vi "SOUR_POW_ALC_MODE_CAT.vi"(0 "VISA IN":refnum<visa-resource-name>, 1 "Port number":i32, 2 "Source Port":string, 5 "error in":errorcluster, 7 "Channel":i32) -> (14 "VISA Out":refnum<visa-resource-name>, 16 "Data":string, 19 "error out":errorcluster)   [LabVIEW 2018, in "PNA-X.lvlib"]
doc: "SOURce<cnum>:POWer<port>:ALC[:MODE]:CATalog?, [src] \n(Read-Write) Returns a list of valid ALC modes for the specified channel and port number. Use the \nreturned values to set SOUR:POW:ALC:MODE. \nParameters \n<cnum> Any existing channel number. If unspecified, value is set to 1 \n<port> Port number of the PNA. If unspecified, value is set to 1. To make settings for \nports that are not simple numbers, use the [src] argument. \n[src] String. (NOT case sensitive). Source port. Optional. Use SOUR:CAT? to \nreturn a list of valid port names. \nWhile this argument can be used to make settings for ALL ports, it is designed \nto access ports that are not simple numbers, such as \"Port 1 Src2\". Otherwise, \nthe <port> argument performs the same function. If both arguments are \nspecified, [src] takes priority. \nExamples SOUR:POW:ALC:MODE:CAT? \nsource2:power2:alc:mode:catalog? \nsource:power:alc:mode:catalog? \"Port 1 Src2\" \nReturn Type Comma-separated list of strings. \nDefault Not applicable"
uses:
  PNA-X.lvlib
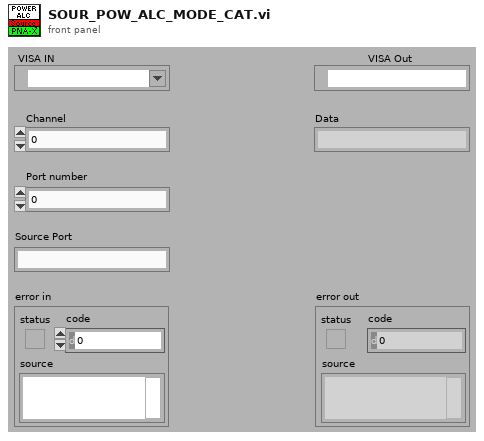
[diagram p1: front panel]
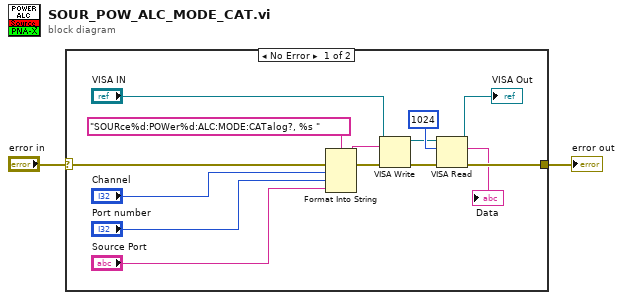
[diagram p0: block diagram]
diagram:
  n1 = case shown="No Error" "error in" {
    selector: "error in" -> [w16 w17]
    tunnel: [w8 w17] -> w1
    frame No Error {
      n2 = Format Into String(format string="SOURce%d:POWer%d:ALC:MODE:CATalog?, %s " ("Cmdline"), error in=w16, "Channel", "Port number", "Source Port") -> (resulting string=w14:string, error out=w15:errorcluster)  [unwired: 1 in]
      n3 = VISA Write(VISA resource name="VISA IN", write buffer=w14, error in (no error)=w15) -> (VISA resource name out=w9:refnum<visa-resource-name>, error out=w11:errorcluster)  [unwired: 1 out]
      n4 = VISA Read(VISA resource name=w9, byte count=1024, error in (no error)=w11) -> (VISA resource name out=→"VISA Out":refnum<visa-resource-name>, read buffer=→"Data":string, error out=w8:errorcluster)  [unwired: 1 out]
    }
    frame Error {
    }
  }
  "error out" <- w1
